vi "Get Default Colors.vi"(0 "Default Row In":string[](array[string]), 7 "Columns":T1[](array[typedef]), 9 "# rows":i32, 11 "DefColors":u32[](array[colorbox])) -> (4 "Default Row Out":string[](array[string]))   [LabVIEW 2020]
uses:
  ColumnSpec.ctl
  ColumnType.ctl
  KTable.xctl
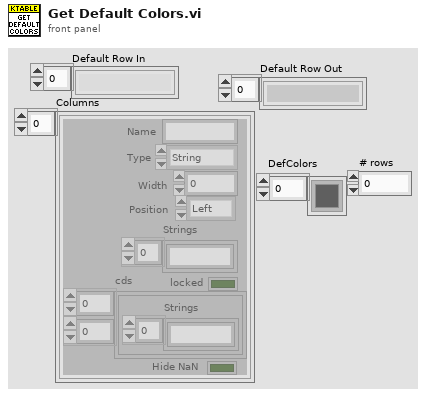
[diagram p1: front panel]
types:
  T1 = typedef "KTable.xctl/ColumnSpec.ctl" = cluster{"Name":string, "Type":T2, "Width":i32, "Strings":string[], "Position":enum16{"Left", "Center", "Right"}, "locked":bool, "cds":cluster{"Strings":string[]}[][], "Hide NaN":bool}
  T2 = typedef "KTable.xctl/ColumnType.ctl" = enum16{"String", "Enum", "Int", "Double", "Boolean", "Ring", "Formula", "Color"}
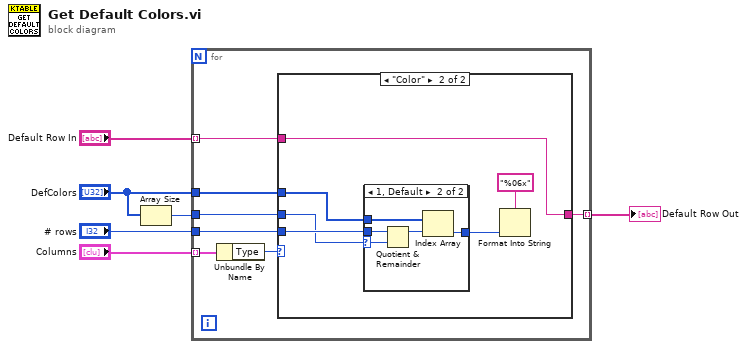
[diagram p0: block diagram]
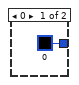
[diagram p3: hidden frame]
diagram:
  n1 = Array Size(array="DefColors") -> (size(s)=w2:i32)
  n2 = for {
    tunnel: "Columns" -> [w13] mode=indexing
    tunnel: "Default Row In" -> [w12] mode=indexing
    tunnel: [w10] -> w6 mode=indexing
    tunnel: "# rows" -> [w9]
    tunnel: "DefColors" -> [w8]
    tunnel: w2 -> [w7]
    n3 = Unbundle By Name(w13) -> ("Type"=w11:T2)
    n4 = case shown="\"Color\"" w11 {
      tunnel: w12 -> [w14 w15]
      tunnel: [w14 w15] -> w10
      tunnel: w9 -> [_ w18]
      tunnel: w8 -> [_ w17]
      tunnel: w7 -> [_ w16]
      frame "String", Default {
      }
      frame "Color" {
        n5 = case shown="1, Default" w16 {
          selector: w16 -> [_ w25]
          tunnel: w17 -> [_ w24]
          tunnel: w18 -> [_ w26]
          tunnel: [u32 0 w22] -> w20
          frame 0 {
          }
          frame 1, Default {
            n6 = Quotient & Remainder(x=w26, y=w25) -> (x-y*floor(x/y)=w23:i32)  [unwired: 1 out]
            n7 = Index Array(array=w24, index=w23) -> (element=w22:u32)
          }
        }
        n8 = Format Into String(format string="%06x", w20) -> ()  [unwired: 2 in, 2 out]
      }
    }
  }
  "Default Row Out" <- w6
